vi "LV SCISDK Get Parameter String.vi"(8 "error in (no error)":errorcluster, 10 "handle":u64, 11 "Path":string) -> (0 "error out":errorcluster, 1 "function return":i32, 2 "handle out":u64, 3 "value":string)   [LabVIEW 2021, in "SciSDK_Labview.lvlib"]
doc: "SCISDKLABVIEW_DLL_API int LV_SCISDK_GetParameterString(char* Path, char* value, void* handle);"
uses:
  SciSDK_Labview.lvlib
  <userlib>/SciSDK_Labview/SciSDK_Labview.dll
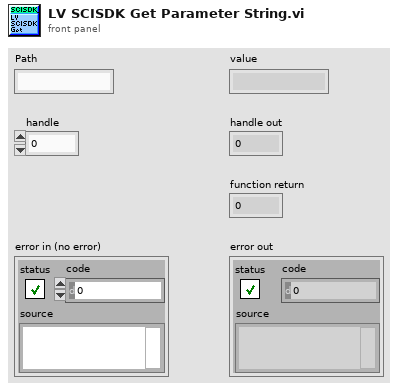
[diagram p1: front panel]
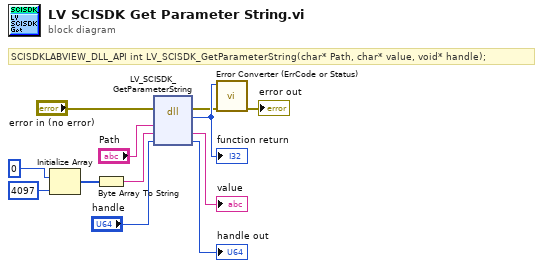
[diagram p0: block diagram]
diagram:
  # "SCISDKLABVIEW_DLL_API int LV_SCISDK_GetParameterString(char* Path, char* value, void* handle);"
  n1 = Initialize Array(u8 0 ("element"), 4097 ("dimension size")) -> (w10:u8[])
  n2 = Byte Array To String(unsigned byte array=w10) -> (string=w9:string)
  n3 = dll-call lib="C:/Program Files/National Instruments/LabVIEW 2021/user.lib/SciSDK_Labview/SciSDK_Labview.*" fn="LV_SCISDK_GetParameterString"(error in="error in (no error)", "Path"="Path", "value"=w9, "handle"="handle") -> (error out=w2:errorcluster, w12:i32, "value"=→"value":string, "handle"=→"handle out":u64)  [unwired: 3 in, 1 out]
  "function return" <- w12
  n4 = call <userlib>:"Error Converter (ErrCode or Status).vi"("error in (no error)"=w2, "error code"=w12) -> ("error out"=→"error out":errorcluster)  [unwired: 9 in]
